vi "WPI_CameraGet Image Appearance Property.vi"(8 "error in (no error)":errorcluster, 9 "Appearance":bool=TRUE, 10 "Prop String":string, 11 "address":string="192.168.0.90") -> (0 "error out":errorcluster, 3 "Value":string)   [LabVIEW 2017]
doc: "This software is licensed. Open the labview\\readme\\WPI Robotics Library Open Source License.txt file for more information."
panel:
  out "Complete Response":string
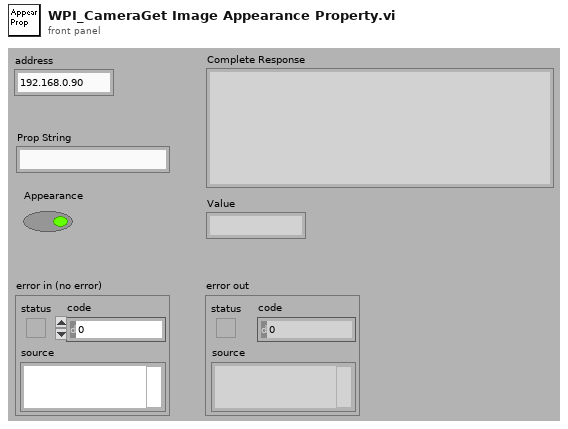
[diagram p1: front panel]
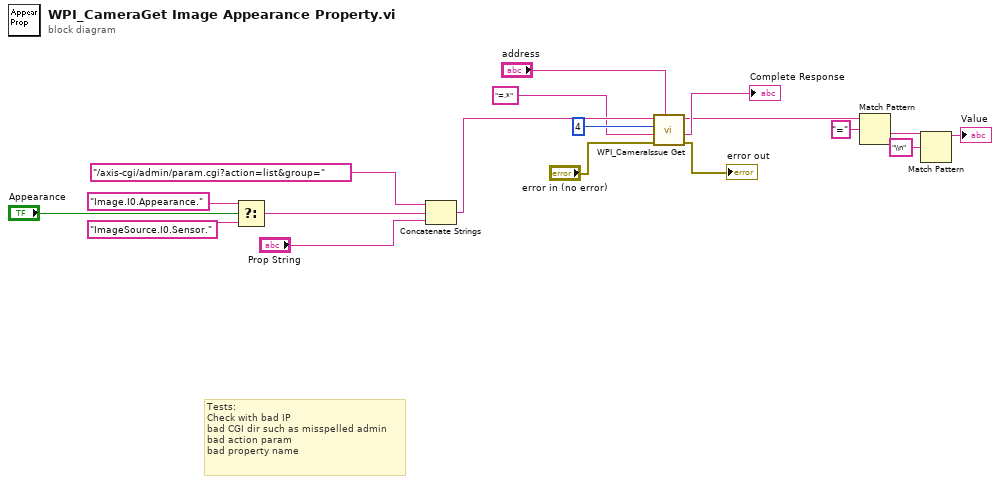
[diagram p0: block diagram]
diagram:
  # "Tests:\nCheck with bad IP\nbad CGI dir such as misspelled admin\nbad action param\nbad property name"
  n1 = Select(t="Image.I0.Appearance.", s="Appearance", f="ImageSource.I0.Sensor.") -> (s? t:f=w2:string)
  n2 = Concatenate Strings("/axis-cgi/admin/param.cgi?action=list&group=", w2, "Prop String") -> (w16:string)
  n3 = call <vilib>:"WPI_CameraIssue Get.vi"("address"="address", "error in (no error)"="error in (no error)", "Regular Expression of text to extract"="=.*", "Number of Lines Expected"=4, "Request"=w16) -> ("error out"=→"error out":errorcluster, "Complete Response"=→"Complete Response":string, "Extracted String"=w10:string)  [unwired: 4 out]
  n4 = Match Pattern(string=w10, regular expression="=") -> (after substring=w8:string)  [unwired: 4 out]
  n5 = Match Pattern(string=w8, regular expression="\\n") -> (before substring=→"Value":string)  [unwired: 4 out]
